vi "format version string.vi"(3 "Version":T1 {"Build Date/Time" format="%<%X\n%x>T"}) -> (1 "Version String":string)   [LabVIEW 2011]
uses:
  Summitek EXT/Miscellaneous/OGAB Version.ctl
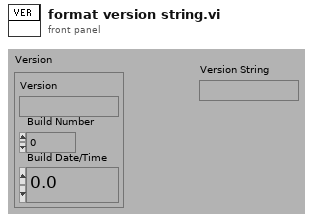
[diagram p1: front panel]
types:
  T1 = typedef "OGAB Version.ctl" = cluster{"Version":string, "Build Number":u32, "Build Date/Time":dbl}
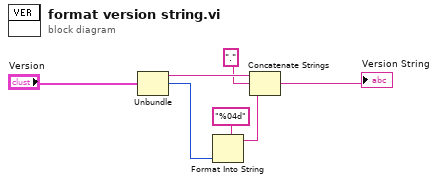
[diagram p0: block diagram]
diagram:
  n1 = Unbundle("Version") -> ("Version"=w7:string, "Build Number"=w4:u32)  [unwired: 1 out]
  n2 = Format Into String(format string="%04d", w4) -> (resulting string=w3:string)  [unwired: 2 in, 1 out]
  n3 = Concatenate Strings(w7, ".", w3) -> (→"Version String":string)
